vi "Register UI Stop Event.vi"(8 "error in":errorcluster, 10 "Stop Button [ref]":refnum<vi>, 11 "Server Stop":refnum<user-event>) -> (0 "error out":errorcluster)   [LabVIEW 2020, in "CancellableMeasurement.lvlib"]
uses:
  CancellableMeasurement.lvlib
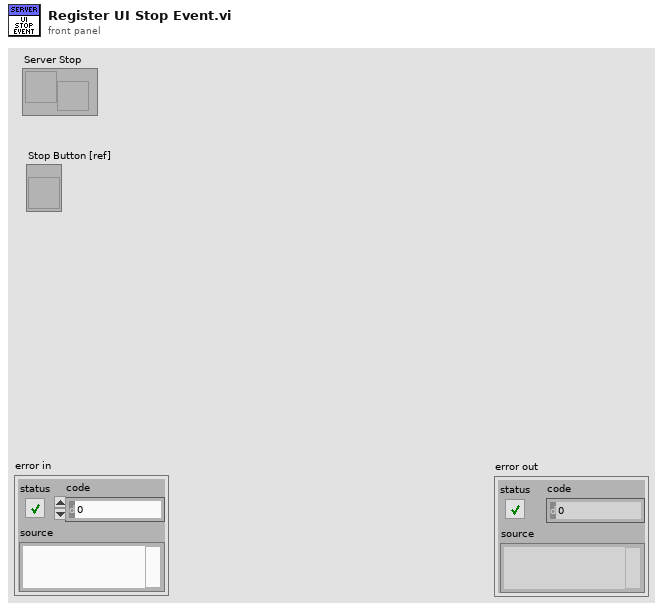
[diagram p1: front panel]
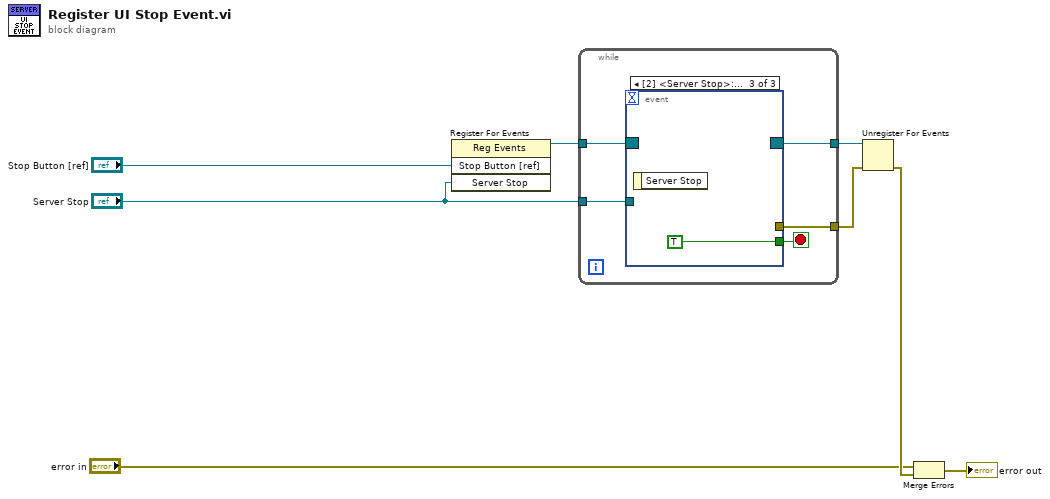
[diagram p0: block diagram]
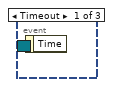
[diagram p2: hidden frame]
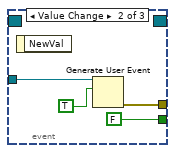
[diagram p3: hidden frame]
diagram:
  n1 = register-events("Stop Button [ref]", "Server Stop") -> (reference out=w8:refnum<event-registration>)  [unwired: 2 in, 1 out]
  n2 = while {
    tunnel: w8 -> [w13]
    tunnel: [w11] -> w7
    tunnel: [w9] -> w6
    tunnel: "Server Stop" -> [w10]
    stop <- w12 stop-if-true
    n3 = event shown="[2] <Server Stop>: User Event" {
      selector: w13 -> [_ _ _]
      dyn-events: [_ _ _] -> w11
      timeout: _ -> [_ _ _]
      tunnel: [_ FALSE TRUE] -> w12
      tunnel: w10 -> [_ w16 _]
      tunnel: [_ w14 _] -> w9
      event Timeout {
        n4 = event-data() -> ()  [unwired: 1 in, 1 out]
      }
      event Value Change {
        n5 = event-data() -> ()  [unwired: 1 in, 1 out]
        n6 = Generate User Event(user event=w16, event data cluster=TRUE ("event data")) -> (error out=w14:errorcluster)  [unwired: 2 in, 1 out]
      }
      event User Event {
        n7 = event-data() -> ()  [unwired: 1 in, 1 out]
      }
    }
  }
  n8 = Unregister For Events(event registration refnum=w7, error in=w6) -> (error out=w5:errorcluster)
  n9 = Merge Errors("error in", w5) -> (→"error out":errorcluster)
